vi "globalvariables.vi"() -> ()   [LabVIEW 2021]
panel:
  out "Peltier Tamb":dbl
  out "Peltier Stop":bool
  out "Peltier Save":bool
  out "Peltier Control Sensor":dbl[](array[numeric])
  out "Peltier Set Power":dbl[](array[numeric])
  out "Peltier Update Rate":i32
  out "Control Mode":i32
  out "Valve Update Rate":i32
  out "Valve Set Temp":dbl[](array[numeric])
  in  "Valve Gains":cluster{"P":dbl, "I":dbl, "D":dbl}[](array[cluster])
  out "Peltier Update":bool[](array[boolean])
  out "Valve Position":dbl[](array[numeric])
  out "Peltier Set Temp":dbl[](array[numeric])
  out "Peltier New Value":bool
  out "Valve New Value":bool
  out "Peltier Control Mode":i16
  out "Valve Control Mode":i16
  out "Sources":i32[](array[numeric])
  out "# of USB DAQ":i32
  out "Calibration Table":dbl[][](array[numeric])
  out "Voltage Limits":dbl[][](array[numeric])
  out "Sensor Descriptions":string[][](array[string])
  out "Sensor Labels":i32[][](array[numeric])
  out "Timer Length":dbl
  out "Path":path
  out "File Name":string
  out "# of ThM":i32
  out "# of sensors":i32
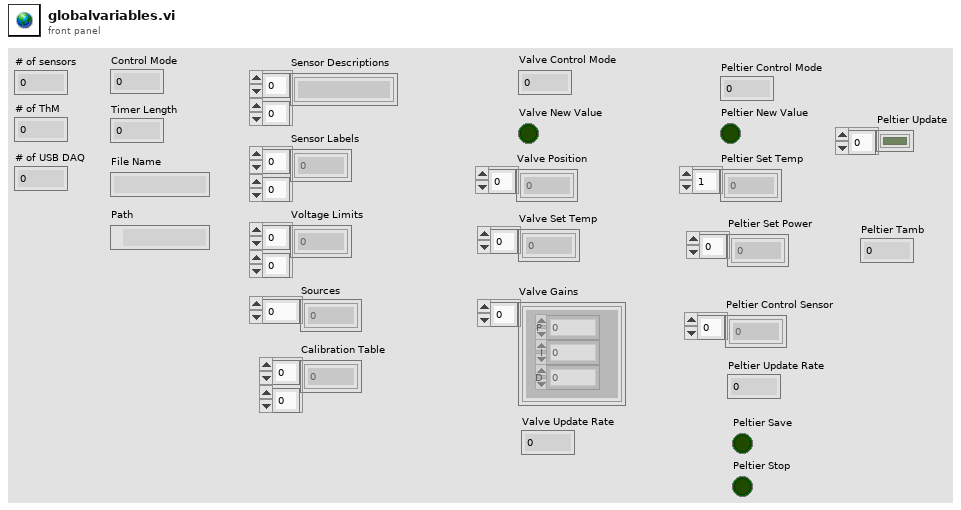
[diagram p1: front panel]
diagram:
